vi "SendBackChannelTrigger.vi"(4 "Custom back channel data":string, 5 "PostEmbedded Data Lines":cluster{"mipiDataType":u8, "Line Data":u8[]}[](array[cluster]), 6 "Image scaling coefficients":dbl[](array[numeric]), 7 "PreEmbedded Data Lines":cluster{"mipiDataType":u8, "Line Data":u8[]}[](array[cluster]), 8 "error in":errorcluster, 10 "Output timestamp (working time)":u64, 11 "rdma session in":refnum<k21>) -> (0 "error out":errorcluster, 3 "rdma session out":refnum<k21>)   [LabVIEW 2021]
uses:
  3be7b388-f881-499e-b1f7-ef9912d54514.vi
  3be7b388-f881-499e-b1f7-ef9912d54514.vi/c7caca0c-161a-4e5d-b028-879c1e2dca2f.vi
  3be7b388-f881-499e-b1f7-ef9912d54514.vi/72e164ce-c078-45d0-ba5f-a1d3dac130e9.vi
  <vilib>/rdma/rdma.llb/RDMA Acquire Send Buffer U8.vi
panel:
  in  "Fault Injection Mode":u8
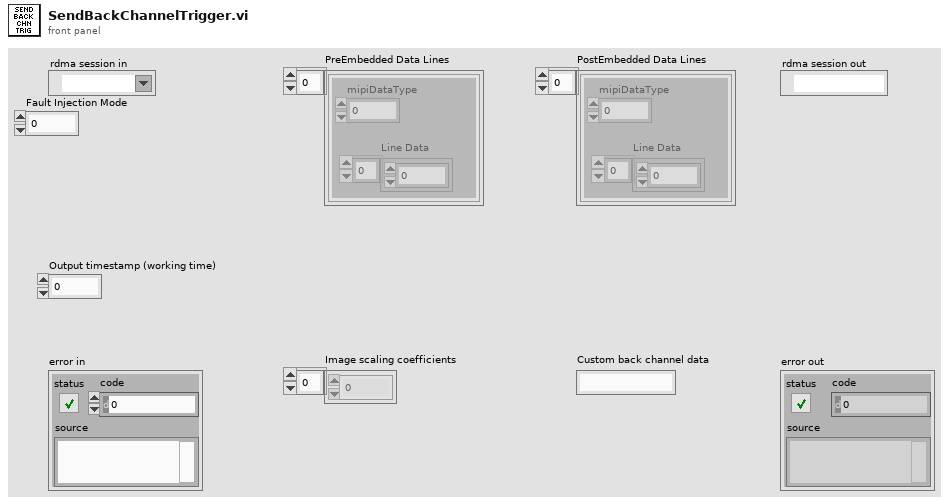
[diagram p1: front panel]
types:
  T1 = enum16{"big-endian, network order", "native, host order", "little-endian"}
  T2 = cluster{"command":u32, "timestampOutput_WorkingTime":u64, "timestampRequested_SystemTime":u64, "imageScalingCoefficientsSize":u32, "preEmbeddedDataTotalSize":u32, "postEmbeddedDataTotalSize":u32, "customBackChannelDataSize":u32, "faultInjectionFlag":u8}
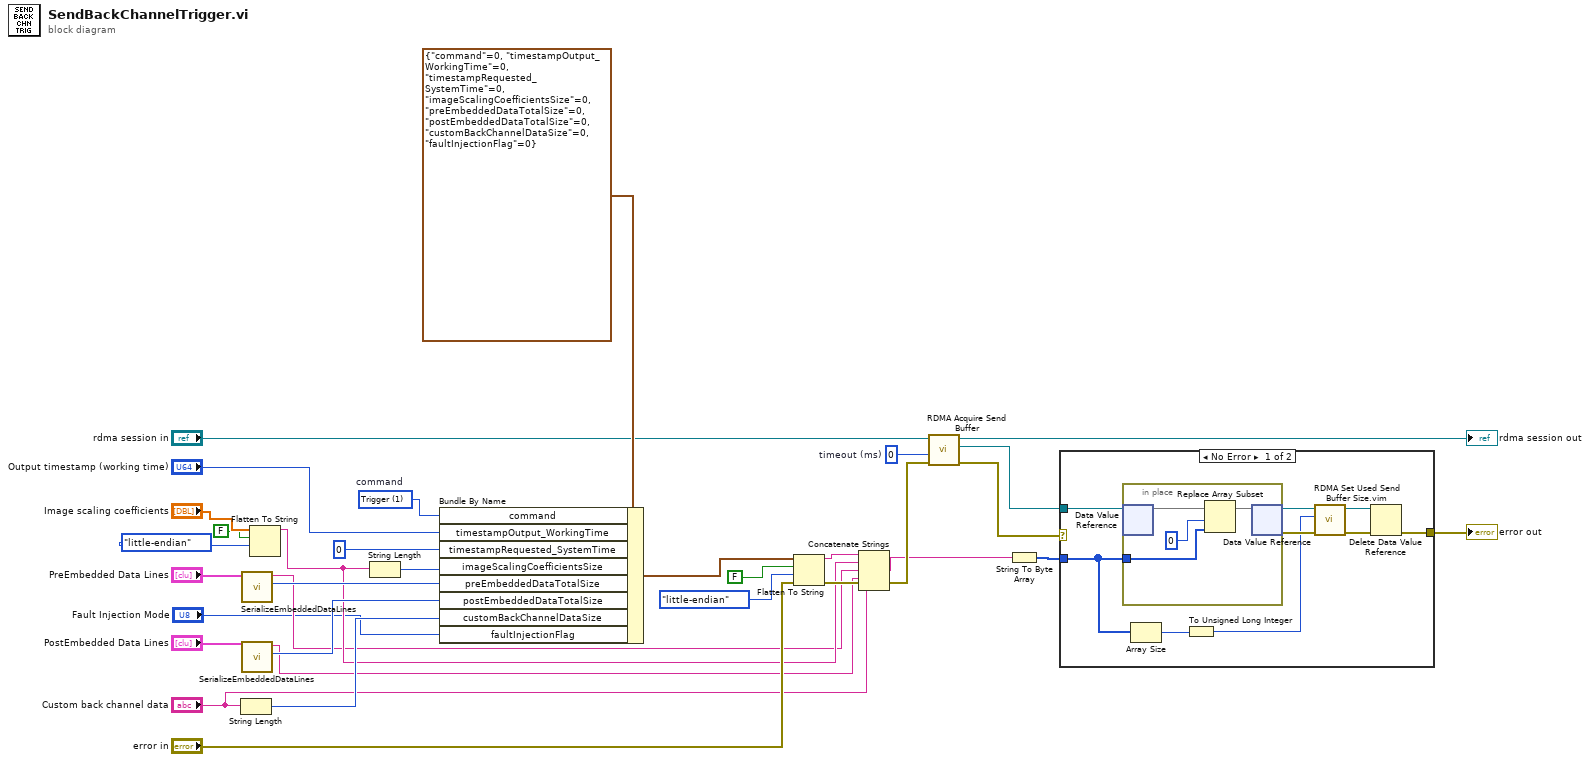
[diagram p0: block diagram]
diagram:
  w12 = u32 1 items=["Trigger"=1]  # command
  w23 = 0  # timeout (ms)
  n1 = String Length(string="Custom back channel data") -> (length=w26:i32)
  n2 = call "SerializeEmbeddedDataLines.vi"("Embedded Data Lines"="PreEmbedded Data Lines") -> ("length"=w25:i32, "Serialized embedded data"=w4:string)  [unwired: 9 in]
  n3 = call "SerializeEmbeddedDataLines.vi"("Embedded Data Lines"="PostEmbedded Data Lines") -> ("length"=w27:i32, "Serialized embedded data"=w3:string)  [unwired: 9 in]
  n4 = Flatten To String(anything="Image scaling coefficients", prepend array or string size? (T)=FALSE, byte order (0:big-endian, network order)=T1."little-endian") -> (data string=w5:string)  [unwired: 1 in, 2 out]
  n5 = String Length(string=w5) -> (length=w8:i32)
  n6 = Bundle By Name(cluster=T2 {"command"=0, "timestampOutput_WorkingTime"=0, "timestampRequested_SystemTime"=0, "imageScalingCoefficientsSize"=0, "preEmbeddedDataTotalSize"=0, "postEmbeddedDataTotalSize"=0, "customBackChannelDataSize"=0, "faultInjectionFlag"=0}, "command"=w12, "timestampOutput_WorkingTime"="Output timestamp (working time)", "timestampRequested_SystemTime"=u64 0, "imageScalingCoefficientsSize"=w8, "preEmbeddedDataTotalSize"=w25, "postEmbeddedDataTotalSize"=w27, "customBackChannelDataSize"=w26, "faultInjectionFlag"="Fault Injection Mode") -> (w19:T2)
  n7 = Flatten To String(anything=w19, prepend array or string size? (T)=FALSE, byte order (0:big-endian, network order)=T1."little-endian", error in (no error)="error in") -> (data string=w7:string, error out=w14:errorcluster)  [unwired: 1 out]
  n8 = Concatenate Strings(w7, w5, w4, w3, "Custom back channel data") -> (w6:string)
  n9 = call-poly <vilib>:"RDMA Acquire Send Buffer.vi"("error in"=w14, "timeout (ms)"=w23, "rdma session in"="rdma session in") -> ("error out"=w22:errorcluster, "edvr"=w20:refnum<data-value>, "rdma session out"=→"rdma session out":refnum<k21>)  [unwired: 6 in]
  n10 = String To Byte Array(string=w6) -> (unsigned byte array=w16:u8[])
  n11 = case shown="No Error" w22 {
    selector: w22 -> [_ w46]
    tunnel: w20 -> [w41 _]
    tunnel: w16 -> [w36 _]
    tunnel: [w33 w46] -> w15
    frame No Error {
      n12 = in-place {
        in-place-border: w36 -> [w44]
        n13 = in-place-dvr #1(w41) -> (w45:u8[])  [unwired: 1 out]
        n14 = Replace Array Subset(array=w45, new element=w44, index=0) -> (w42:u8[])
        n15 = in-place-dvr #1(w42) -> (w40:refnum<data-value>, w38:errorcluster)
      }
      n16 = Array Size(array=w36) -> (size(s)=w35:i32)
      n17 = To Unsigned Long Integer(number=w35) -> (unsigned 32bit integer=w34:u32)
      n18 = call "RDMA Set Used Send Buffer Size.vim"("error in"=w38, "used send buffer size"=w34, "edvr in"=w40) -> ("error out"=w37:errorcluster, "edvr out"=w39:refnum<data-value>)  [unwired: 7 in]
      n19 = Delete Data Value Reference(data value reference=w39, error in=w37) -> (error out=w33:errorcluster)  [unwired: 1 out]
    }
    frame Error {
    }
  }
  "error out" <- w15
